vi "Test_5 objects.vi"() -> ()   [LabVIEW 2017]
panel:
  in  "Gp A pieces (n,d)":i32[][](array[numeric])=array10000x2[20000 elements]
  out "Posterior":dbl[][](graph)=[[0.06686866999999999, 0.08124426000000001, 0.06493801, 0.03670863, 0.011140430000000002], [0.08111895, 0.09855810000000001, 0.07877685000000001, 0.044531549999999996, 0.01351455], [0.06205023, 0.07538994, 0.060258690000000004, 0.03406347, 0.01033767], [0.03403664, 0.04135392, 0.03305392, 0.01868496, 0.005670560000000001], [0.012225509999999998, 0.01485378, 0.011872530000000001, 0.006711389999999999, 0.00203679]]
  out "Posterior":dbl[][](array[numeric])
  out "A likelihoods, p(n,d|A)":dbl[][](graph)=[[0.06686866999999999, 0.08124426000000001, 0.06493801, 0.03670863, 0.011140430000000002], [0.08111895, 0.09855810000000001, 0.07877685000000001, 0.044531549999999996, 0.01351455], [0.06205023, 0.07538994, 0.060258690000000004, 0.03406347, 0.01033767], [0.03403664, 0.04135392, 0.03305392, 0.01868496, 0.005670560000000001], [0.012225509999999998, 0.01485378, 0.011872530000000001, 0.006711389999999999, 0.00203679]]
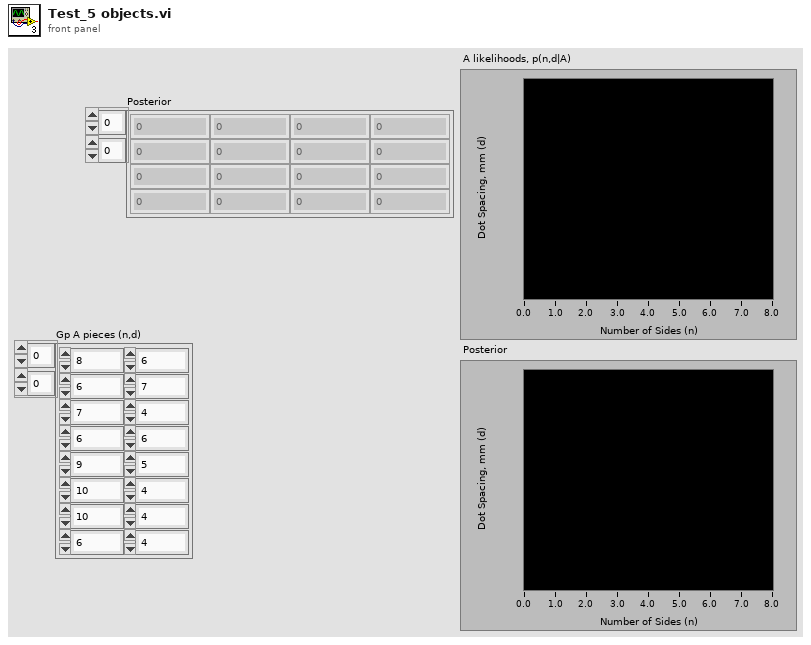
[diagram p1: front panel]
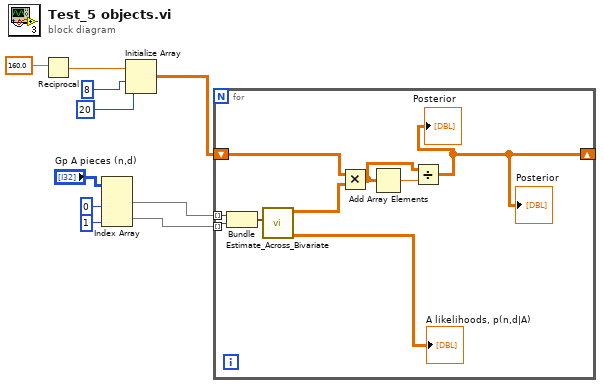
[diagram p0: block diagram]
diagram:
  n1 = Reciprocal(x=160.0) -> (1/x=w9:dbl)
  n2 = Index Array(array="Gp A pieces (n,d)", index (col) #1=0 ("disabled index (col)"), index (col) #2=1 ("index (col)")) -> (element #1=w3:i32[], element #2=w4:i32[])  [unwired: 2 in]
  n3 = Initialize Array(w9, 8 ("dimension size"), 20 ("dimension size")) -> (w6:dbl[][])
  n4 = for {
    tunnel: w4 -> [w19] mode=indexing
    tunnel: w3 -> [w18] mode=indexing
    shift-right: [w11] -> _
    shift-left: w6 -> [w14]
    n5 = Bundle(w18, w19) -> (w17:cluster{i32, i32})  [unwired: 1 in]
    n6 = call "Estimate_Across_Bivariate.vi"("Data"=w17) -> ("A likelihoods, p(n,d|A)"=→"A likelihoods, p(n,d|A)":dbl[][], "Marginalize Across SD's"=w15:dbl[][])  [unwired: 7 in, 2 out]
    n7 = Multiply(x=w14, y=w15) -> (x*y=w12:dbl[][])
    n8 = Add Array Elements(numeric array=w12) -> (sum=w13:dbl)
    n9 = Divide(x=w12, y=w13) -> (x/y=w11:dbl[][])
    "Posterior" <- w11
    "Posterior" <- w11
  }
